vi "Handle Error.vi"(8 "error in (no error)":errorcluster, 11 "Tesla Factory Tester in":refnum<class "Tesla Factory Tester.lvclass">) -> (0 "error out":errorcluster, 2 "stop actor?":bool=TRUE, 3 "Tesla Factory Tester out":refnum<class "Tesla Factory Tester.lvclass">)   [LabVIEW 2013, in "Tesla Factory Tester.lvlib" / "Tesla Factory Tester.lvclass"]
doc: "(<B>Filename</B>: Actor Framework.lvlib:Actor.lvclass:Handle Error.vi)\n\nDefines how the actor handles an error that occurred while processing a message.\n\nBy default, this method does nothing except stop the actor. This method also treats error code 43 (coming from <B>error in</B>) as a sign that the actor shut down normally. In this situation, the Handle Error method does not return the error on <B>error out</B>, meaning the actor's caller will not receive it. All other error codes will be returned on <B>error out</B>.\n\nA descendant class may override this method to change this behavior."
uses:
  Tesla Factory Tester.lvclass
  <vilib>/ActorFramework/Actor/Actor.lvclass
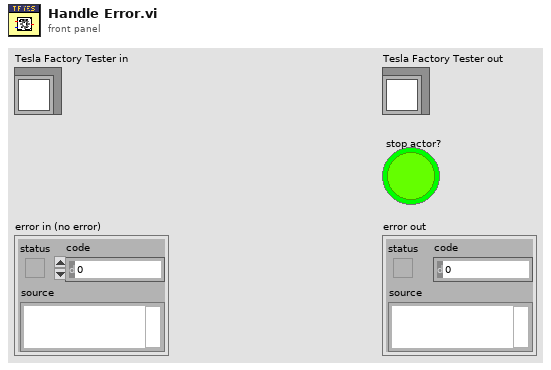
[diagram p1: front panel]
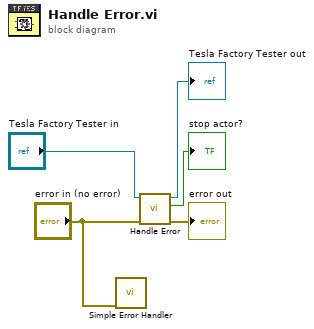
[diagram p0: block diagram]
diagram:
  n1 = call <vilib>:"Simple Error Handler.vi"("error in (no error)"="error in (no error)") -> ()  [unwired: 4 in, 5 out]
  n2 = call-parent "Handle Error.vi"("error in (no error)"="error in (no error)", "Actor in"="Tesla Factory Tester in") -> ("error out"=→"error out":errorcluster, "stop actor?"=→"stop actor?":bool, "Actor out"=→"Tesla Factory Tester out":refnum<class "Tesla Factory Tester.lvclass">)  [unwired: 7 in]
